vi "calibrate trap data V2.vi"(4 "Offset File step size":dbl, 5 "delta frequency":dbl, 6 "Dynamic offset update":bool, 7 "Offsets":cluster{"T1X offset":dbl[], "T2X offset":dbl[]}, 8 "T2 calibration":T1 {"offset_y (mV)" format="%#_2g"; "kappa_y (pN/nm)" min=0.0 step=0.001 format="%#_2g"; "alpha_y (nm/V)" step=10.0 format="%#_3g"; "kappa_x (pN/nm)" min=0.0 step=0.001 format="%#_2g"; "offset_x (mV)" format="%#_2g"; "alpha_x (nm/V)" step=10.0 format="%#_3g"}, 9 "T2":dbl[](array[numeric]), 10 "T1 calibration":T1 {"offset_y (mV)" format="%#_2g"; "kappa_y (pN/nm)" min=0.0 step=0.001 format="%#_2g"; "alpha_y (nm/V)" step=10.0 format="%#_3g"; "kappa_x (pN/nm)" min=0.0 step=0.001 format="%#_2g"; "offset_x (mV)" format="%#_2g"; "alpha_x (nm/V)" step=10.0 format="%#_3g"}, 11 "T1":dbl[](array[numeric])) -> (0 "T2 force (pN)":dbl[](array[numeric]), 1 "T2 position (nm)":dbl[](array[numeric]), 2 "T1 force (pN)":dbl[](array[numeric]), 3 "T1 position (nm)":dbl[](array[numeric]))   [LabVIEW 2014]
panel:
  in  "T3 calibration":T1 {"offset_y (mV)" format="%#_2g"; "kappa_y (pN/nm)" min=0.0 step=0.001 format="%#_2g"; "alpha_y (nm/V)" step=10.0 format="%#_3g"; "kappa_x (pN/nm)" min=0.0 step=0.001 format="%#_2g"; "offset_x (mV)" format="%#_2g"; "alpha_x (nm/V)" step=10.0 format="%#_3g"}
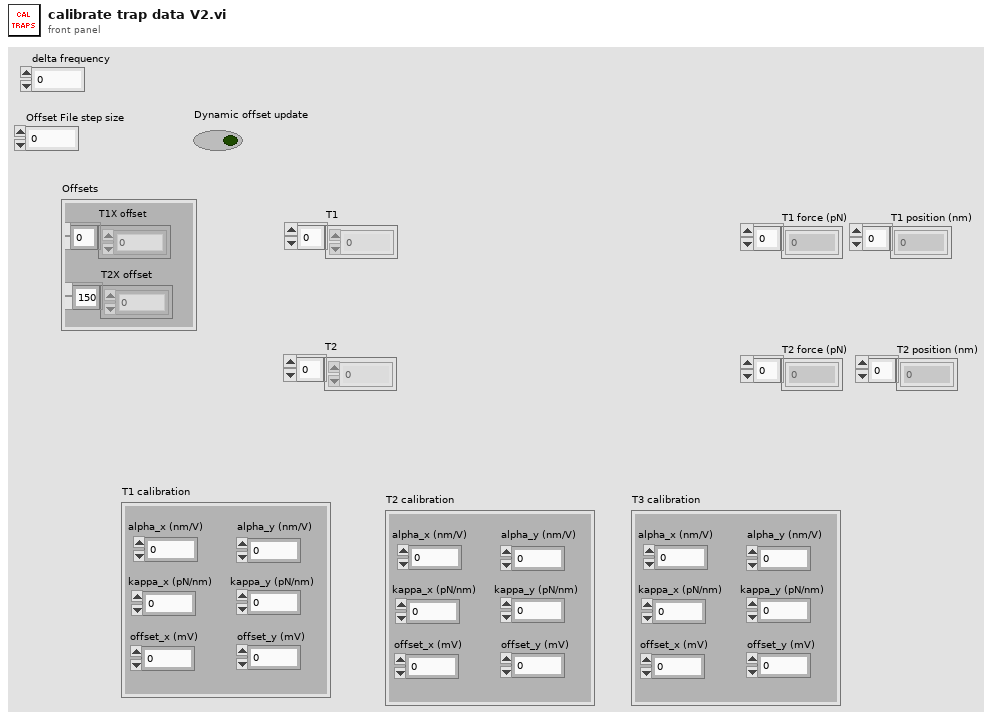
[diagram p1: front panel]
types:
  T1 = cluster{"alpha_x (nm/V)":dbl, "offset_x (mV)":dbl, "kappa_x (pN/nm)":dbl, "alpha_y (nm/V)":dbl, "kappa_y (pN/nm)":dbl, "offset_y (mV)":dbl}
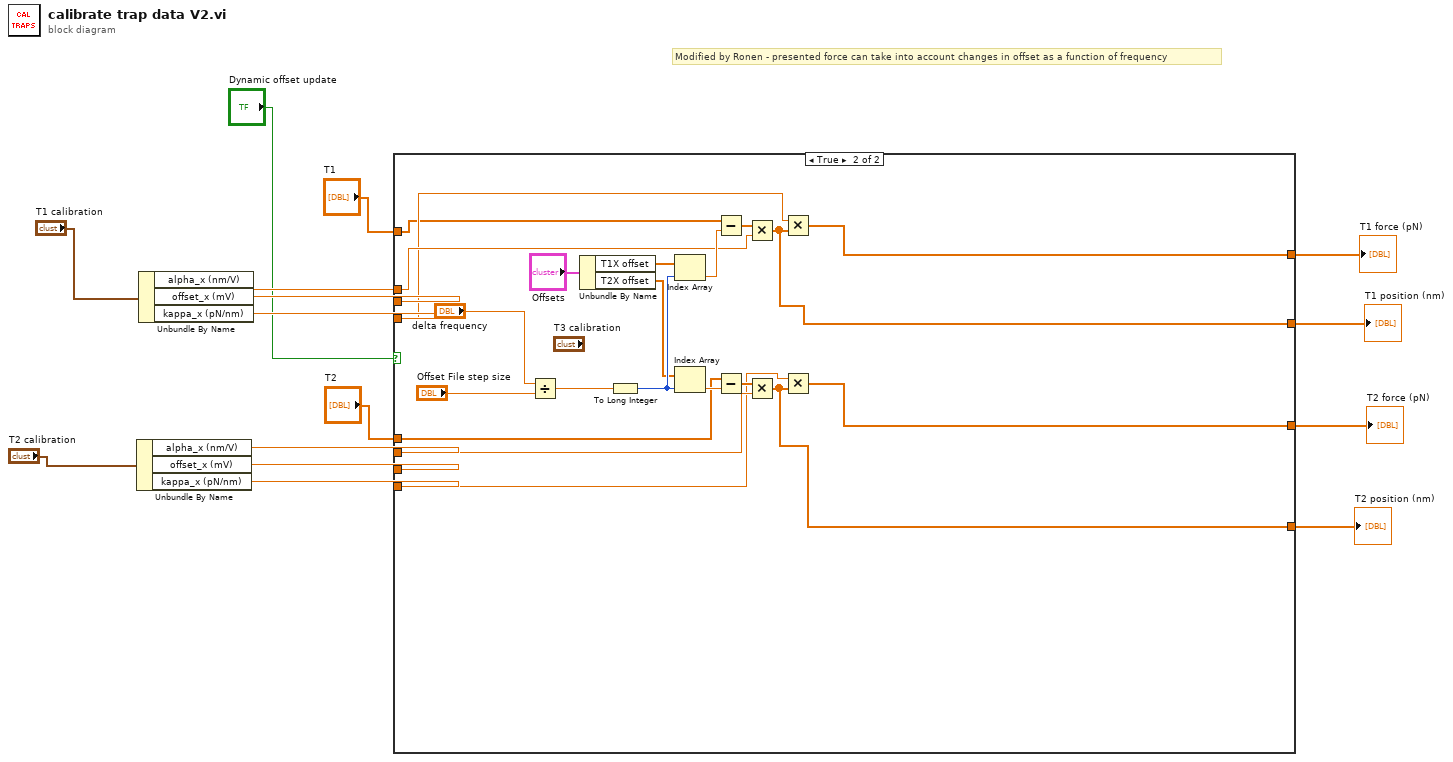
[diagram p0: block diagram]
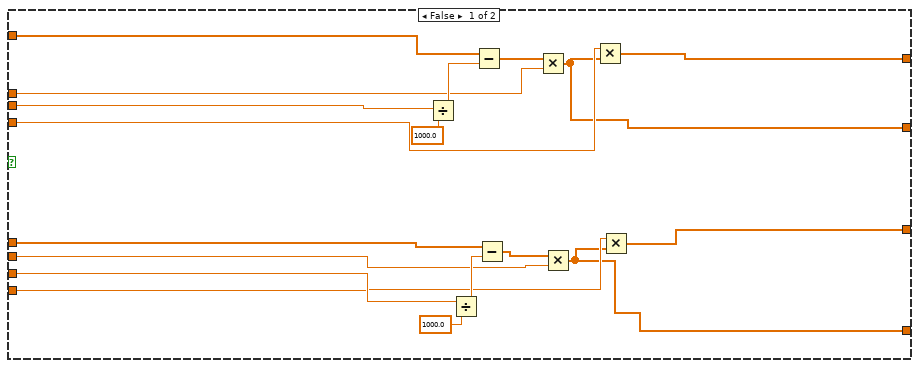
[diagram p2: hidden frame]
diagram:
  # "Modified by Ronen - presented force can take into account changes in offset as a function of frequency"
  n1 = Unbundle By Name("T2 calibration") -> ("alpha_x (nm/V)"=w12:dbl, "offset_x (mV)"=w14:dbl, "kappa_x (pN/nm)"=w10:dbl)
  n2 = Unbundle By Name("T1 calibration") -> ("alpha_x (nm/V)"=w13:dbl, "offset_x (mV)"=w15:dbl, "kappa_x (pN/nm)"=w11:dbl)
  n3 = case shown="True" "Dynamic offset update" {
    tunnel: w15 -> [w27 _]
    tunnel: w14 -> [w26 _]
    tunnel: w13 -> [w25 w44]
    tunnel: w12 -> [w24 w41]
    tunnel: w11 -> [w23 w43]
    tunnel: w10 -> [w22 w40]
    tunnel: "T2" -> [w21 w39]
    tunnel: "T1" -> [w20 w38]
    tunnel: [w19 w34] -> w6
    tunnel: [w18 w35] -> w5
    tunnel: [w17 w36] -> w4
    tunnel: [w16 w37] -> w3
    frame False {
      n4 = Divide(x=w27, y=1000.0) -> (x/y=w31:dbl)
      n5 = Divide(x=w26, y=1000.0) -> (x/y=w30:dbl)
      n6 = Subtract(x=w20, y=w31) -> (x-y=w29:dbl[])
      n7 = Subtract(x=w21, y=w30) -> (x-y=w28:dbl[])
      n8 = Multiply(x=w29, y=w25) -> (x*y=w17:dbl[])
      n9 = Multiply(x=w28, y=w24) -> (x*y=w19:dbl[])
      n10 = Multiply(x=w23, y=w17) -> (x*y=w16:dbl[])
      n11 = Multiply(x=w22, y=w19) -> (x*y=w18:dbl[])
    }
    frame True {
      n12 = Divide(x="delta frequency", y="Offset File step size") -> (x/y=w50:dbl)
      n13 = Unbundle By Name("Offsets") -> ("T1X offset"=w46:dbl[], "T2X offset"=w47:dbl[])
      n14 = To Long Integer(number=w50) -> (32bit integer=w48:i32)
      n15 = Index Array(array=w46, index=w48) -> (element=w45:dbl)
      n16 = Index Array(array=w47, index=w48) -> (element=w42:dbl)
      n17 = Subtract(x=w38, y=w45) -> (x-y=w54:dbl[])
      n18 = Subtract(x=w39, y=w42) -> (x-y=w53:dbl[])
      n19 = Multiply(x=w54, y=w44) -> (x*y=w36:dbl[])
      n20 = Multiply(x=w53, y=w41) -> (x*y=w34:dbl[])
      n21 = Multiply(x=w43, y=w36) -> (x*y=w37:dbl[])
      n22 = Multiply(x=w40, y=w34) -> (x*y=w35:dbl[])
    }
  }
  "T1 force (pN)" <- w3
  "T1 position (nm)" <- w4
  "T2 force (pN)" <- w5
  "T2 position (nm)" <- w6
